vi "BigDataFits_U16_FGV.vi"(8 "InError":errorcluster caption="entrée d'erreur (pas d'erreur)", 9 "ClustBigFilFits":T1={"file (use dialog)"=path "D:/DATA/Imatest.fits", "Type de données"=enum."I16 (signed integer 16bit)", "Commentaire"="", "naxis1"=0, "naxis2"=0, "naxis3"=1, "Exptime"=1.0}, 10 "entier 16 bits":u16[][](array[numeric]), 11 "Énum":T3) -> (0 "sortie d'erreur":errorcluster)   [LabVIEW 2020]
doc: "Permet la sauvegarde des données sous forme de U16. \n Unsigned 16-bit and 32-bit integers are supported by subtracting an offset from the raw pixel values (e.g., 32768 (2**15) is subtracted from each unsigned 16-bit integer pixel value to shift the values into the range of a signed 16-bit integer) before writing them to the FITS file. This offset is then added (BZERO) to the pixels when reading the FITS image to restore the original values."
uses:
  BigDataFits.ctl
  ClustBigFilFits.ctl
  DataTyp_Header.ctl
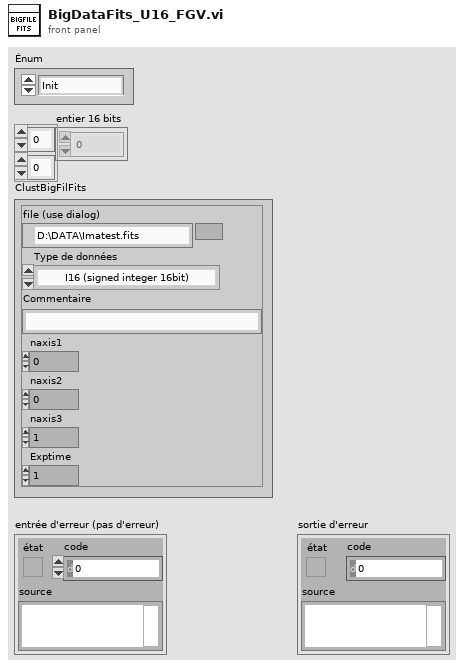
[diagram p1: front panel]
types:
  T1 = typedef "ClustBigFilFits.ctl" = cluster{"file (use dialog)":path, "Type de données":T2, "Commentaire":string, "naxis1":i32, "naxis2":i32, "naxis3":i32, "Exptime":sgl}
  T2 = typedef "DataTyp_Header.ctl" = enum16{"U8 (unsigned integer 8bit)", "I16 (signed integer 16bit)", "U16 (unsigned integer 16 bit)", "I32 (signed integer 32bit)", "U32 (unsigned integer 32 bit)", "SGL (float 32bit)", "DBL(float 64bit)", "complex (2xfloat 64bit)"}
  T3 = typedef "BigDataFits.ctl" = enum16{"Init", "WritHeader", "WritData", "Close"}
  T4 = enum16{"open", "replace", "create", "open or create", "replace or create", "replace or create with confirmation"}
  T5 = enum16{"big-endian, network order", "native, host order", "little-endian"}
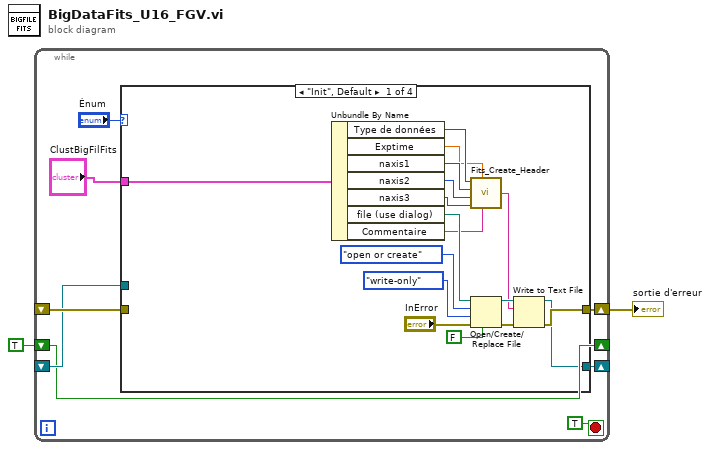
[diagram p0: block diagram]
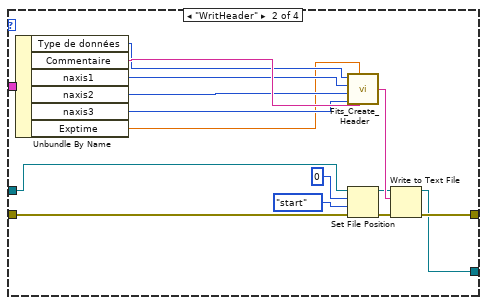
[diagram p2: hidden frame]
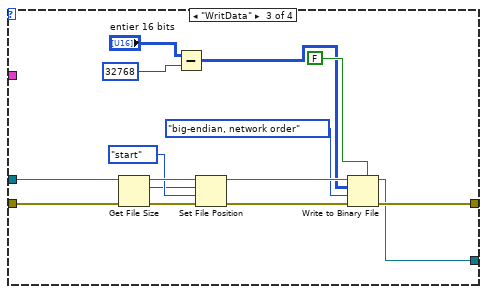
[diagram p3: hidden frame]
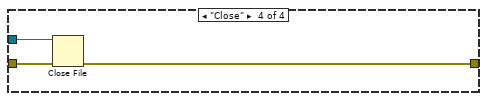
[diagram p4: hidden frame]
diagram:
  n1 = while {
    shift-right: [w4] -> _
    shift-left: TRUE -> [w4]
    shift-right: [w7] -> _
    shift-left: _ -> [w5]
    shift-right: [w8] -> w2
    shift-left: _ -> [w6]
    stop <- TRUE stop-if-true
    n2 = case shown="\"Init\", Default" "Énum" {
      tunnel: [w21 w42 w48 w60] -> w8
      tunnel: [w20 w41 w47 _] -> w7
      tunnel: w6 -> [_ w37 w50 w61]
      tunnel: w5 -> [_ w36 w49 w59]
      tunnel: "ClustBigFilFits" -> [w19 w34 _ _]
      frame "Init", Default {
        n3 = Unbundle By Name(w19) -> ("Type de données"=w14:T2, "Exptime"=w12:sgl, "naxis1"=w17:i32, "naxis2"=w16:i32, "naxis3"=w15:i32, "file (use dialog)"=w18:path, "Commentaire"=w13:string)
        n4 = call "Fits_Create_Header.vi"("Commentaire"=w13, "Exptim"=w12, "naxis3"=w15, "naxis2"=w16, "naxis1"=w17, "Type de données"=w14) -> ("FITS header"=w22:string)
        n5 = Open/Create/Replace File(file path (use dialog)=w18, error in="InError", operation (0:open)=T4."open or create" ("opération (0 : open)"), access (0:read/write)=enum16{"read/write", "read-only", "write-only"}."write-only" ("accès (0 : read/write)"), disable buffering (F)=FALSE) -> (refnum out=w23:refnum<file>, error out=w24:errorcluster)  [unwired: 1 in, 1 out]
        n6 = Write to Text File(file (use dialog)=w23, text=w22, error in=w24) -> (refnum out=w20:refnum<file>, error out=w21:errorcluster)  [unwired: 1 in, 1 out]
      }
      frame "WritHeader" {
        n7 = Unbundle By Name(w34) -> ("Type de données"=w29:T2, "Commentaire"=w33:string, "naxis1"=w30:i32, "naxis2"=w31:i32, "naxis3"=w32:i32, "Exptime"=w28:sgl)
        n8 = call "Fits_Create_Header.vi"("Commentaire"=w33, "Exptim"=w28, "naxis3"=w32, "naxis2"=w31, "naxis1"=w30, "Type de données"=w29) -> ("FITS header"=w43:string)
        n9 = Set File Position(offset (in bytes) (0)=i64 0 ("offset (en octets) (0)"), refnum=w36, from (0:start)=enum16{"start", "end", "current"}."start" ("à partir de (0 : start)"), error in=w37) -> (refnum out=w35:refnum<file>, error out=w38:errorcluster)
        n10 = Write to Text File(file (use dialog)=w35, text=w43, error in=w38) -> (refnum out=w41:refnum<file>, error out=w42:errorcluster)  [unwired: 1 in, 1 out]
      }
      frame "WritData" {
        n11 = Get File Size(file=w49, error in=w50) -> (refnum out=w58:refnum<file>, size (in bytes)=w55:i64, 0:w56:errorcluster)
        n12 = Subtract(x="entier 16 bits", y=u16 32768) -> (x-y=w45:u16[][])
        n13 = Set File Position(offset (in bytes) (0)=w55, refnum=w58, from (0:start)=enum16{"start", "end", "current"}."start" ("à partir de (0 : start)"), error in=w56) -> (refnum out=w53:refnum<file>, error out=w54:errorcluster)
        n14 = Write to Binary File(file (use dialog)=w53, data=w45, error in=w54, 5:FALSE ("ajouter une taille de tableau ou de chaîne ? (V)"), 9:T5."big-endian, network order" ("ordre des octets (0 : big-Endian, network order)")) -> (refnum out=w47:refnum<file>, error out=w48:errorcluster)  [unwired: 1 in, 1 out]
      }
      frame "Close" {
        n15 = Close File(refnum=w59, error in=w61) -> (error out=w60:errorcluster)  [unwired: 1 out]
      }
    }
  }
  "sortie d'erreur" <- w2
